vi "To String.vi"(8 "error in (no error)":errorcluster, 11 "JSON Basic Type in":refnum<class "JSON Basic Type.lvclass">) -> (0 "error out":errorcluster, 2 "String":string, 3 "JSON Basic Type out":refnum<class "JSON Basic Type.lvclass">)   [LabVIEW 2017, in "JSON Basic Type.lvclass"]
uses:
  JSON Basic Type.lvclass
  JSON Datatype/JSON Datatype.lvclass
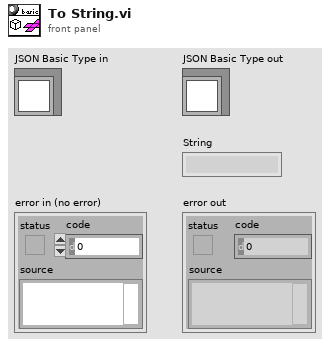
[diagram p1: front panel]
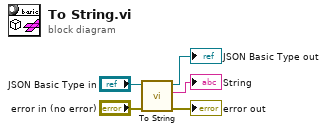
[diagram p0: block diagram]
diagram:
  n1 = call-parent "To String.vi"("error in (no error)"="error in (no error)", "JSON Datatype in"="JSON Basic Type in") -> ("error out"=→"error out":errorcluster, "String"=→"String":string, "JSON Datatype out"=→"JSON Basic Type out":refnum<class "JSON Basic Type.lvclass">)  [unwired: 7 in]
